vi "Lifetime.vi"(0 "N":i32=1) -> (1 "N+1":i32, 2 "N-1":i32)   [LabVIEW 2009, in "HB_BaseClass_Examples.lvlib"]
doc: "Demo of data lifetime."
uses:
  HB_BaseClass_Examples.lvlib
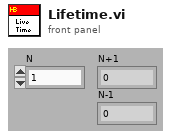
[diagram p1: front panel]
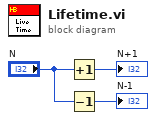
[diagram p0: block diagram]
diagram:
  n1 = Increment(x="N") -> (x+1=→"N+1":i32)
  n2 = Decrement(x="N") -> (x-1=→"N-1":i32)
